vi "ConvertTextBasedCodeToLabVIEW_AddMethodContentToBdOfClassMethod.vi"(8 "error in (no error)":errorcluster, 9 "MethodContent":string, 10 "MethodName":string, 11 "ClassPath(*.lvclass)":path) -> (0 "error out":errorcluster)   [LabVIEW 2014]
doc: "This VI creates Methods in a class."
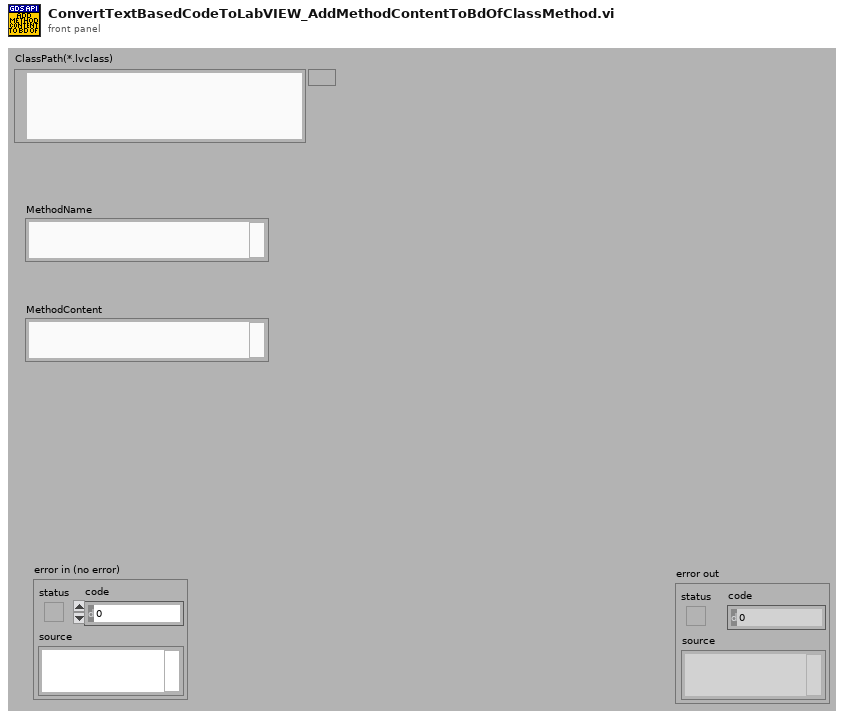
[diagram p1: front panel]
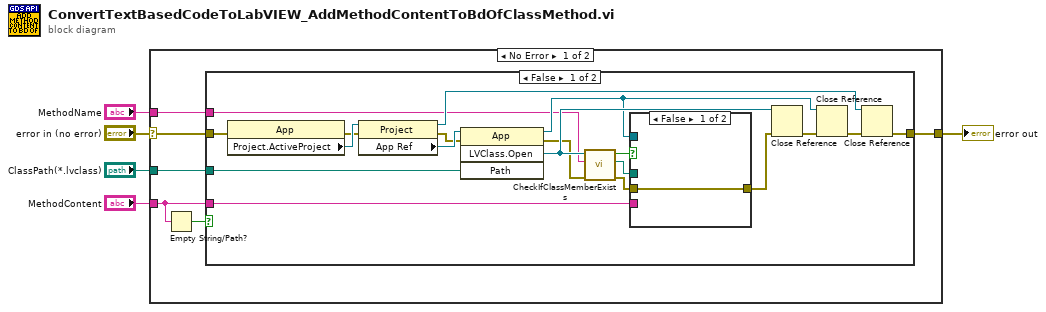
[diagram p0: block diagram]
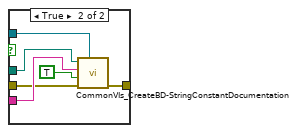
[diagram p2: hidden frame]
diagram:
  n1 = case shown="No Error" "error in (no error)" {
    selector: "error in (no error)" -> [w9 w39]
    tunnel: "ClassPath(*.lvclass)" -> [w11 _]
    tunnel: [w10 w39] -> w4
    tunnel: "MethodContent" -> [w8 _]
    tunnel: "MethodName" -> [w6 _]
    frame No Error {
      n2 = Empty String/Path?(string/path=w8) -> (empty?=w7:bool)
      n3 = case shown="False" w7 {
        tunnel: w11 -> [w30 _]
        tunnel: [w23 w38] -> w10
        tunnel: w9 -> [w18 w38]
        tunnel: w8 -> [w17 _]
        tunnel: w6 -> [w14 _]
        frame False {
          n4 = property class="App"(error in=w18) -> (error out=w26:errorcluster, "Project.ActiveProject"=w29:refnum<vi>)  [unwired: 1 in, 1 out]
          n5 = property class="Project"(reference=w29, error in=w26) -> (reference out=w20:refnum<vi>, error out=w27:errorcluster, "App Ref"=w28:refnum<vi>)
          n6 = invoke class="App" method="LVClass.Open"(reference=w28, error in=w27, "Path"=w30) -> (reference out=w19:refnum<vi>, error out=w21:errorcluster, "LVClass.Open"=w22:refnum<vi>)  [unwired: 1 in, 1 out]
          n7 = call <resource>:"CheckIfClassMemberExists.vi"("error in (no error)"=w21, "MethodName"=w14, "LVClassLibrary in"=w22) -> ("error out"=w16:errorcluster, "Path"=w13:path, "Exists"=w12:bool)  [unwired: 6 in]
          n8 = case shown="False" w12 {
            tunnel: w19 -> [_ w37]
            tunnel: w17 -> [_ w36]
            tunnel: w16 -> [w31 w35]
            tunnel: [w31 w34] -> w15
            tunnel: w13 -> [_ w32]
            frame False {
            }
            frame True {
              n9 = call <resource>:"CommonVIs_CreateBD-StringConstantDocumentation.vi"("App"=w37, "error in (no error)"=w35, "Remove extra prefixed spaces on every row but keep indentation"=TRUE ("Remove extar prefixed spaces on every row but keep indentation"), "Documentation"=w36, "VI Ref/Vi Path"=w32) -> ("error out"=w34:errorcluster)  [unwired: 6 in]
            }
          }
          n10 = Close Reference(reference=w22, error in (no error)=w15) -> (error out=w25:errorcluster)
          n11 = Close Reference(reference=w19, error in (no error)=w25) -> (error out=w24:errorcluster)
          n12 = Close Reference(reference=w20, error in (no error)=w24) -> (error out=w23:errorcluster)
        }
        frame True {
        }
      }
    }
    frame Error {
    }
  }
  "error out" <- w4
